vi "CCSDS Unflatten.vi"(8 "error in (no error)":errorcluster, 11 "CCSDS Packet in":string) -> (0 "error out":errorcluster, 2 "CCSDS Header":T1 {"SeqFlags" format="%02b"; "Version" format="%03b"}, 3 "Remaining Data out":string)   [LabVIEW 2018, in "TCPServer.lvlib"]
uses:
  TCPServer.lvlib
  TypeDefs/CCSDS.ctl
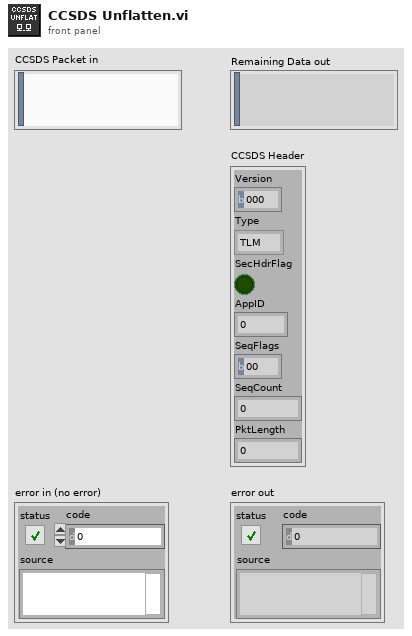
[diagram p1: front panel]
types:
  T1 = typedef "TCPServer.lvlib/CCSDS.ctl" = cluster{"Version":u8, "Type":enum8{"TLM", "CMD"}, "SecHdrFlag":bool, "AppID":u16, "SeqFlags":u8, "SeqCount":u16, "PktLength":u16}
  T2 = cluster{"HDR_TYPE":u16, "HDR_SEQ":u16, "HDR_LENGTH":u16}
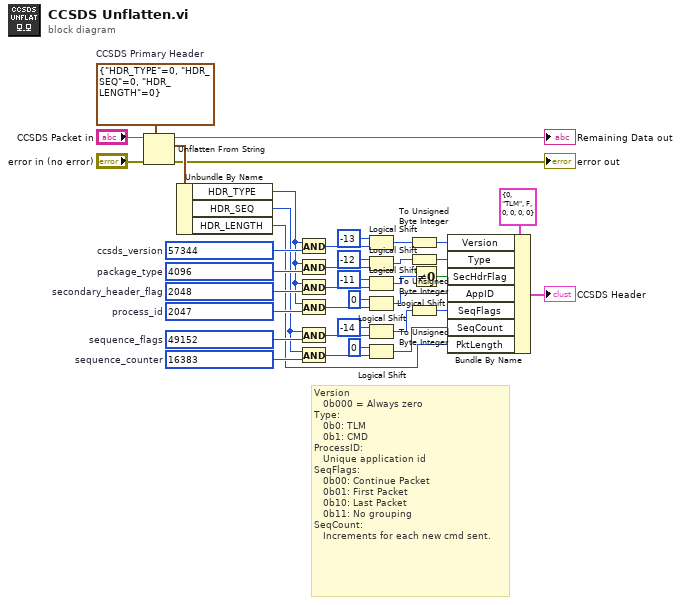
[diagram p0: block diagram]
diagram:
  w17 = u16 16383  # sequence_counter
  w13 = u16 49152  # sequence_flags
  w19 = u16 2047  # process_id
  w26 = u16 2048  # secondary_header_flag
  w30 = u16 4096  # package_type
  w36 = u16 57344  # ccsds_version
  w37 = T2 {"HDR_TYPE"=0, "HDR_SEQ"=0, "HDR_LENGTH"=0}  # CCSDS Primary Header
  # "Version\n   0b000 = Always zero\nType:\n   0b0: TLM\n   0b1: CMD\nProcessID:\n   Unique application id\nSeqFlags:\n   0b00: Continue Packet\n   0b01: First Packet\n   0b10: Last Packet\n   0b11: No grouping\nSeqCount:\n   Increments for each new cmd sent."
  n1 = Unflatten From String(type=w37, binary string="CCSDS Packet in", error in (no error)="error in (no error)") -> (rest of the binary string=→"Remaining Data out":string, value=w6:T2, error out=→"error out":errorcluster)  [unwired: 2 in]
  n2 = Unbundle By Name(w6) -> ("HDR_TYPE"=w5:u16, "HDR_SEQ"=w4:u16, "HDR_LENGTH"=w3:u16)
  n3 = And(x=w5, y=w36) -> (x .and. y?=w35:u16)
  n4 = And(x=w5, y=w30) -> (x .and. y?=w31:u16)
  n5 = And(x=w5, y=w26) -> (x .and. y?=w25:u16)
  n6 = And(x=w5, y=w19) -> (x .and. y?=w20:u16)
  n7 = And(x=w4, y=w13) -> (x .and. y?=w14:u16)
  n8 = And(x=w4, y=w17) -> (x .and. y?=w16:u16)
  n9 = Logical Shift(y=i16 -13, x=w35) -> (x << y=w33:u16)
  n10 = Logical Shift(y=i16 -12, x=w31) -> (x << y=w29:u16)
  n11 = Logical Shift(y=i16 -11, x=w25) -> (x << y=w23:u16)
  n12 = Logical Shift(y=i16 0, x=w20) -> (x << y=w18:u16)
  n13 = Logical Shift(y=i16 -14, x=w14) -> (x << y=w11:u16)
  n14 = Logical Shift(y=i16 0, x=w16) -> (x << y=w10:u16)
  n15 = To Unsigned Byte Integer(number=w33) -> (unsigned 8bit integer=w28:u8)
  n16 = To Unsigned Byte Integer(number=w29) -> (unsigned 8bit integer=w27:u8)
  n17 = To Unsigned Byte Integer(number=w11) -> (unsigned 8bit integer=w9:u8)
  n18 = Not Equal To 0?(x=w23) -> (x != 0?=w22:bool)
  n19 = Bundle By Name(cluster=T1 {"Version"=0, "Type"=enum."TLM", "SecHdrFlag"=FALSE, "AppID"=0, "SeqFlags"=0, "SeqCount"=0, "PktLength"=0} ("CCSDS Primary Header"), "Version"=w28, "Type"=w27, "SecHdrFlag"=w22, "AppID"=w18, "SeqFlags"=w9, "SeqCount"=w10, "PktLength"=w3) -> (→"CCSDS Header":T1)
